vi "Measurement.GetProtectedEventsRegistration.vi"(8 "error in (no error)":errorcluster, 11 "Measurement in":refnum<class "Measurement.lvclass">) -> (0 "error out":errorcluster, 2 "Measurement Protected Events":refnum<event-registration>, 3 "Measurement out":refnum<class "Measurement.lvclass">)   [LabVIEW 2017, in "Measurement.lvclass"]
uses:
  Measurement.lvclass
  Typedefs/ProtectedEvents--Cluster.ctl
  Typedefs/ProtectedEvents--Measurement.Begin.ctl
  Typedefs/ProtectedEvents--Measurement.Pause.ctl
  Typedefs/ProtectedEvents--Measurement.End.ctl
  Typedefs/ProtectedEvents--Measurement.Uninitialize.ctl
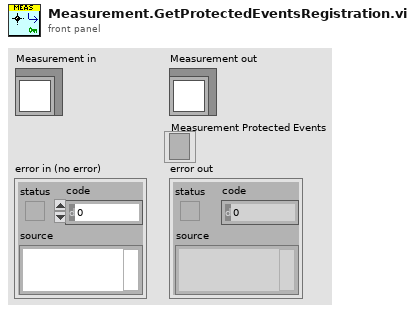
[diagram p1: front panel]
types:
  T1 = typedef "Measurement.lvclass/ProtectedEvents--Cluster.ctl" = cluster{"Initialize":refnum<user-event>, "Begin":refnum<user-event>, "Pause":refnum<user-event>, "End":refnum<user-event>, "Uninitialize":refnum<user-event>}
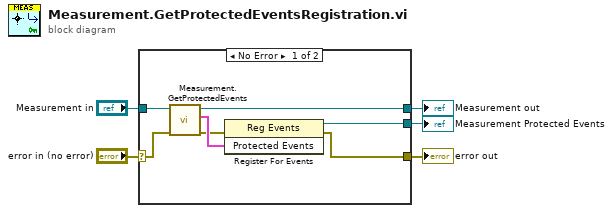
[diagram p0: block diagram]
diagram:
  n1 = case shown="No Error" "error in (no error)" {
    selector: "error in (no error)" -> [w11 w14]
    tunnel: [w8 w14] -> w4
    tunnel: [w7 w13] -> w2
    tunnel: "Measurement in" -> [w12 w13]
    tunnel: [w6 _] -> w1
    frame No Error {
      n2 = call "Measurement.GetProtectedEvents.vi"("error in (no error)"=w11, "Measurement in"=w12) -> ("error out"=w9:errorcluster, "Protected Events"=w10:T1, "Measurement out"=w7:refnum<class "Measurement.lvclass">)  [unwired: 7 in]
      n3 = register-events(error in=w9, w10) -> (reference out=w6:refnum<event-registration>, error out=w8:errorcluster)  [unwired: 1 in]
    }
    frame Error {
    }
  }
  "error out" <- w4
  "Measurement out" <- w2
  "Measurement Protected Events" <- w1
